vi "complementaryfilter.vi"() -> ()   [LabVIEW 2017]
uses:
  <vilib>/myRIO/Common/Instrument Driver Framework/myRIO v1.0/Encoder/typedefs/Encoder Signal Mode.ctl
  <vilib>/myRIO/Instrument Drivers/Onboard IO/Encoder/typedefs/Encoder Reference.ctl
  <vilib>/myRIO/Common/Instrument Driver Framework/Utilities/typedefs/myRIO Generic Hardware Reference.ctl
  <vilib>/myRIO/Common/Instrument Driver Framework/Utilities/typedefs/Hardware Version Enum.ctl
  <vilib>/myRIO/Common/Instrument Driver Framework/Utilities/typedefs/myRIO v1.0 Reference.ctl
  <vilib>/myRIO/Common/Instrument Driver Framework/Utilities/typedefs/Generic FPGA Reference.ctl
  <vilib>/myRIO/Common/Instrument Driver Framework/myRIO v1.0/Encoder/typedefs/Encoder Channels Enum.ctl
  <vilib>/myRIO/Common/Instrument Driver Framework/myRIO v1.0/Encoder/typedefs/Encoder Configuration v1.0.ctl
  <vilib>/userdefined/High Color/nirio_resource_hc.ctl
  <vilib>/myRIO/Common/Instrument Driver Framework/Utilities/vis/Is FPGA Ref Available.vi
  <vilib>/myRIO/Common/Instrument Driver Framework/myRIO v1.0/Encoder/vis/myRIO v1.1 Open Encoder.vi
  <vilib>/myRIO/Instrument Drivers/Onboard IO/Encoder/vis/Read.vi
  <vilib>/myRIO/Common/Instrument Driver Framework/myRIO v1.0/UART/vis/myRIO v1.0 Close UART.vi
  <vilib>/myRIO/Common/Instrument Driver Framework/Utilities/vis/Validate Channels.vi
  <vilib>/myRIO/Common/Instrument Driver Framework/myRIO v1.0/Encoder/vis/myRIO v1.0 Reserve Encoder.vi
  <vilib>/myRIO/Common/Instrument Driver Framework/myRIO v1.0/Encoder/vis/myRIO v1.0 Build MUX Configuration Encoder.vi
  <vilib>/myRIO/Common/Instrument Driver Framework/myRIO v1.0/Resource Manager/vis/myRIO v1.0 Reserve Channel List.vi
  <vilib>/myRIO/Common/Instrument Driver Framework/myRIO v1.0/Resource Manager/vis/myRIO v1.0 Create Configuration List.vi
  <vilib>/myRIO/Common/Instrument Driver Framework/myRIO v1.0/Resource Manager/vis/myRIO v1.0 Reserve Channel.vi
  <vilib>/myRIO/Common/Instrument Driver Framework/myRIO v1.0/Resource Manager/vis/myRIO v1.0 Unreserve Channel.vi
  <vilib>/myRIO/Common/Instrument Driver Framework/myRIO v1.0/Resource Manager/vis/myRIO v1.0 Build Mutex Name.vi
  <vilib>/myRIO/Common/Instrument Driver Framework/Utilities/vis/FPGA Ref Manager.vi
  <vilib>/myRIO/Common/Instrument Driver Framework/myRIO v1.0/myRIO v1.0 Reset FPGA.vi
  <vilib>/myRIO/Common/Instrument Driver Framework/myRIO v1.0/IRQ/vis/myRIO v1.0 IRQ Info FGV.vi
  <vilib>/myRIO/Common/Instrument Driver Framework/myRIO v1.0/IRQ/vis/myRIO v1.0 Timer IRQ Info FGV.vi
  <vilib>/myRIO/Common/Instrument Driver Framework/myRIO v1.0/IRQ/vis/myRIO v1.0 ISR Agent.vi
  <vilib>/Utility/VariantDataType/GetNumericInfo.vi
  <vilib>/Utility/error.llb/Error Cluster From Error Code.vi
  <vilib>/myRIO/Common/Instrument Driver Framework/myRIO v1.0/myRIO v1.1 Open.vi
  <vilib>/myRIO/Common/Instrument Driver Framework/Utilities/vis/IO Manager.vi
  <vilib>/myRIO/Common/Instrument Driver Framework/Utilities/vis/Configuration Manager.vi
  <vilib>/myRIO/Common/Instrument Driver Framework/myRIO v1.0/Resource Manager/vis/myRIO v1.0 Configure IO.vi
  <vilib>/myRIO/Common/Instrument Driver Framework/myRIO v1.0/myRIO v1.0 Close.vi
  <vilib>/myRIO/Common/Instrument Driver Framework/myRIO v1.0/Encoder/vis/myRIO v1.0 Configure Encoder.vi
  <vilib>/myRIO/Common/Instrument Driver Framework/myRIO v1.0/Encoder/vis/myRIO v1.0 Read Encoder.vi
  <vilib>/addons/control/pid/pid.llb/PID (DBL).vi
  <vilib>/myRIO/Express VI/Onboard IO/Encoder/Encoder Express VI.xnode
  <vilib>/myRIO/Instrument Drivers/Onboard IO/Encoder/vis/myRIO Encoder Open.xnode
  <vilib>/myRIO/Common/Instrument Driver Framework/myRIO v1.0/Encoder/typedefs/Encoder Count Direction Enum.ctl
  <vilib>/addons/control/pid/NI_PID_pid.lvlib
  <vilib>/myRIO/Instrument Drivers/Onboard IO/Encoder/Encoder.lvlib
  <vilib>/Analysis/NI_AALPro.lvlib
  <vilib>/robotics/Navigation/shared/WorldMap/OccupancyGridWorldMap/NI_Robotics_OccupancyGridWorldMap.lvclass
  <vilib>/myRIO/Instrument Drivers/Utilities/Utilities.lvlib
panel:
  out "x-y":dbl
  out "angle offset":dbl
  out "latest notification":dbl
  in  "stop 3":bool
  out "string":string
  out "Waveform Chart":cluster{"roll":dbl, "pitch":dbl, "yaw":dbl}(graph)
  out "yaw 2":dbl(graph)
  in  "port":refnum<visa-resource-name>="ASRL2::INSTR"
  out "XY Graph 2":cluster{dbl[], dbl[]}(graph)
  in  "stop 2":bool
  in  "Resolution":dbl=50.0
  out "Intensity Graph":dbl[][](graph)
  out "Frequency":u32=10
  in  "curPos":cluster{"x":i32, "y":i32}
  in  "endPos":cluster{"x":i32, "y":i32}={"x"=0, "y"=6}
  out "path":cluster{"X":i32, "Y":i32}[](array[cluster])
  out "Setpoint B":dbl(slide)=1.3993520911950799 scale=-10.0..10.0
  out "Setpoint A":dbl(slide)=0.6006479088049201 scale=-10.0..10.0
  out "PID B":T1(graph)={"Setpoint"=1.3993520911950799, "output"=0.10115092019020398, "dx/dt"=1.4}
  out "PID A":T1(graph)={"Setpoint"=0.6006479088049201, "output"=0.05446764760463431, "dx/dt"=0.7407999999999447}
  out "OUTPUT A":dbl(slide)=0.7407999999999447 scale=-10.0..10.0
  out "OUTPUT B":dbl(slide)=1.4 scale=-10.0..10.0
  in  "stop":bool
  in  "PID gains":T2={"proportional gain (Kc)"=0.05, "integral time (Ti, min)"=0.05, "derivative time (Td, min)"=0.0} {"derivative time (Td, min)" format="%.3f"; "integral time (Ti, min)" format="%.3f"; "proportional gain (Kc)" format="%.3f"}
  out "XY Graph":cluster{"X":dbl, "Y":dbl}[](graph)=[{"X"=3.638988671509065, "Y"=989.3451951487937}, {"X"=3.4680482195157727, "Y"=989.91873657972}]
  in  "Angle":dbl(slide) scale=-360.0..360.0
  in  "Speed":dbl(slide) scale=-10.0..10.0
  out "X, Y, BEARING 2":cluster{dbl, dbl, dbl}
  out "Final X, Y, BEARING":cluster{dbl, dbl, dbl}
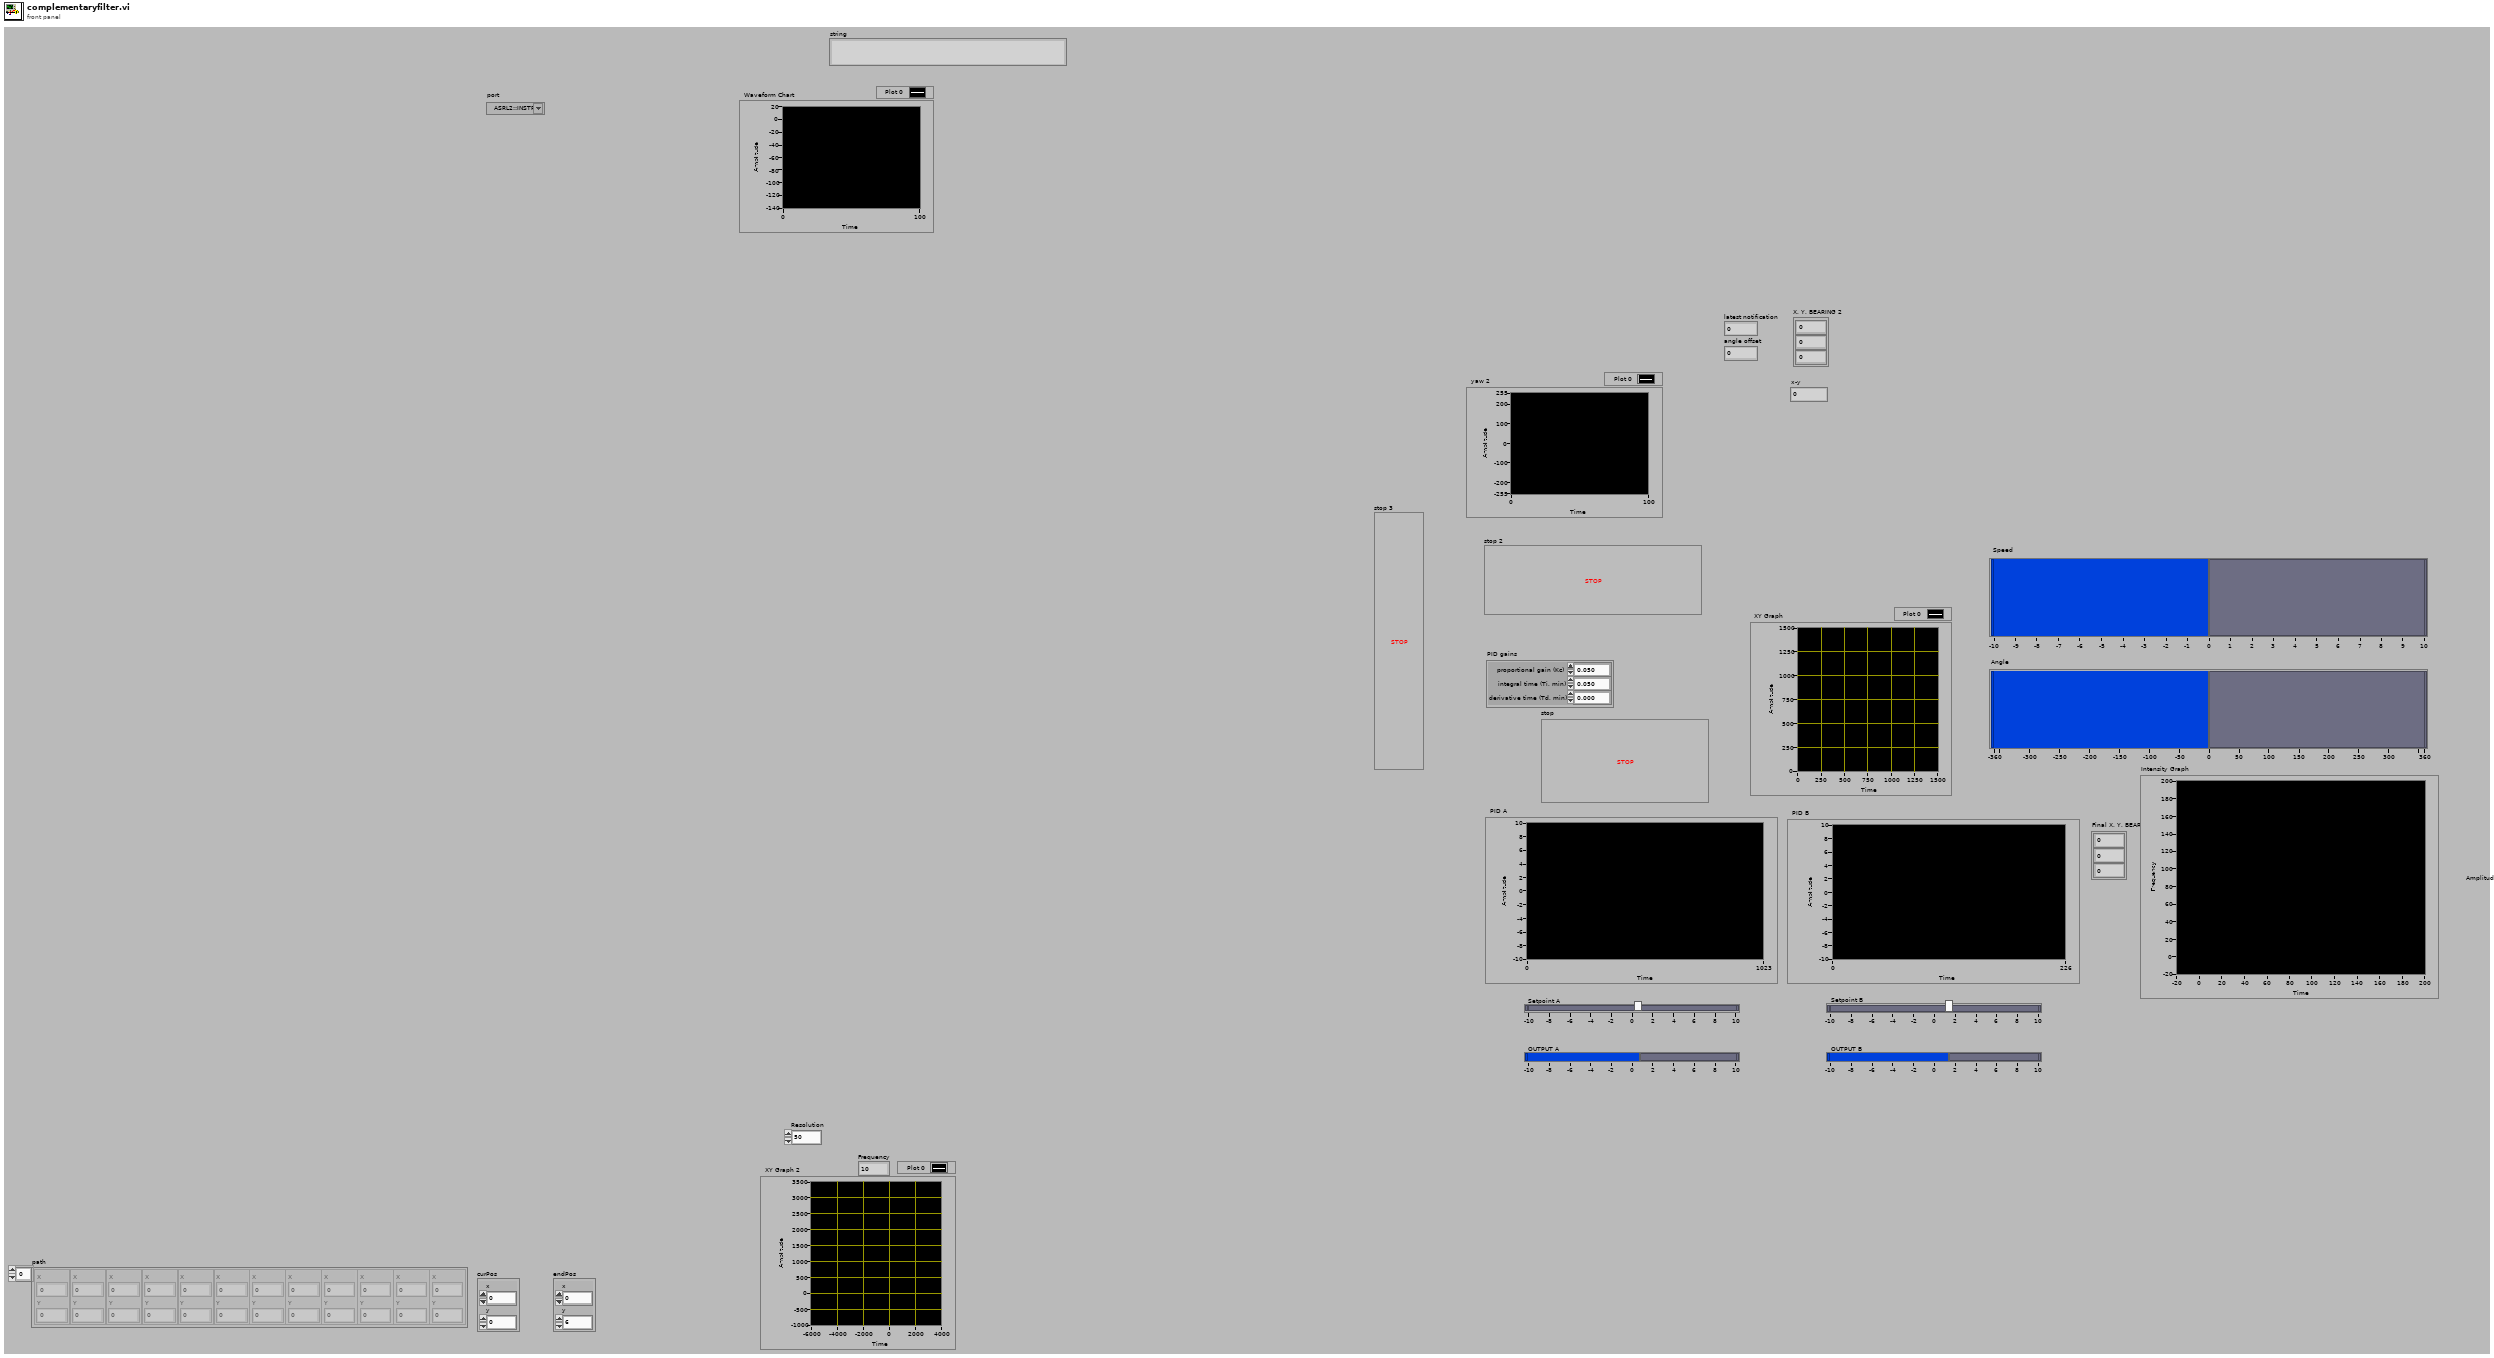
[diagram p1: front panel]
types:
  T1 = cluster{"Setpoint":dbl, "output":dbl, "dx/dt":dbl}
  T2 = cluster{"proportional gain (Kc)":dbl, "integral time (Ti, min)":dbl, "derivative time (Td, min)":dbl}
  T3 = typedef "LidarPoint.ctl" = cluster{"X":dbl, "Y":dbl}
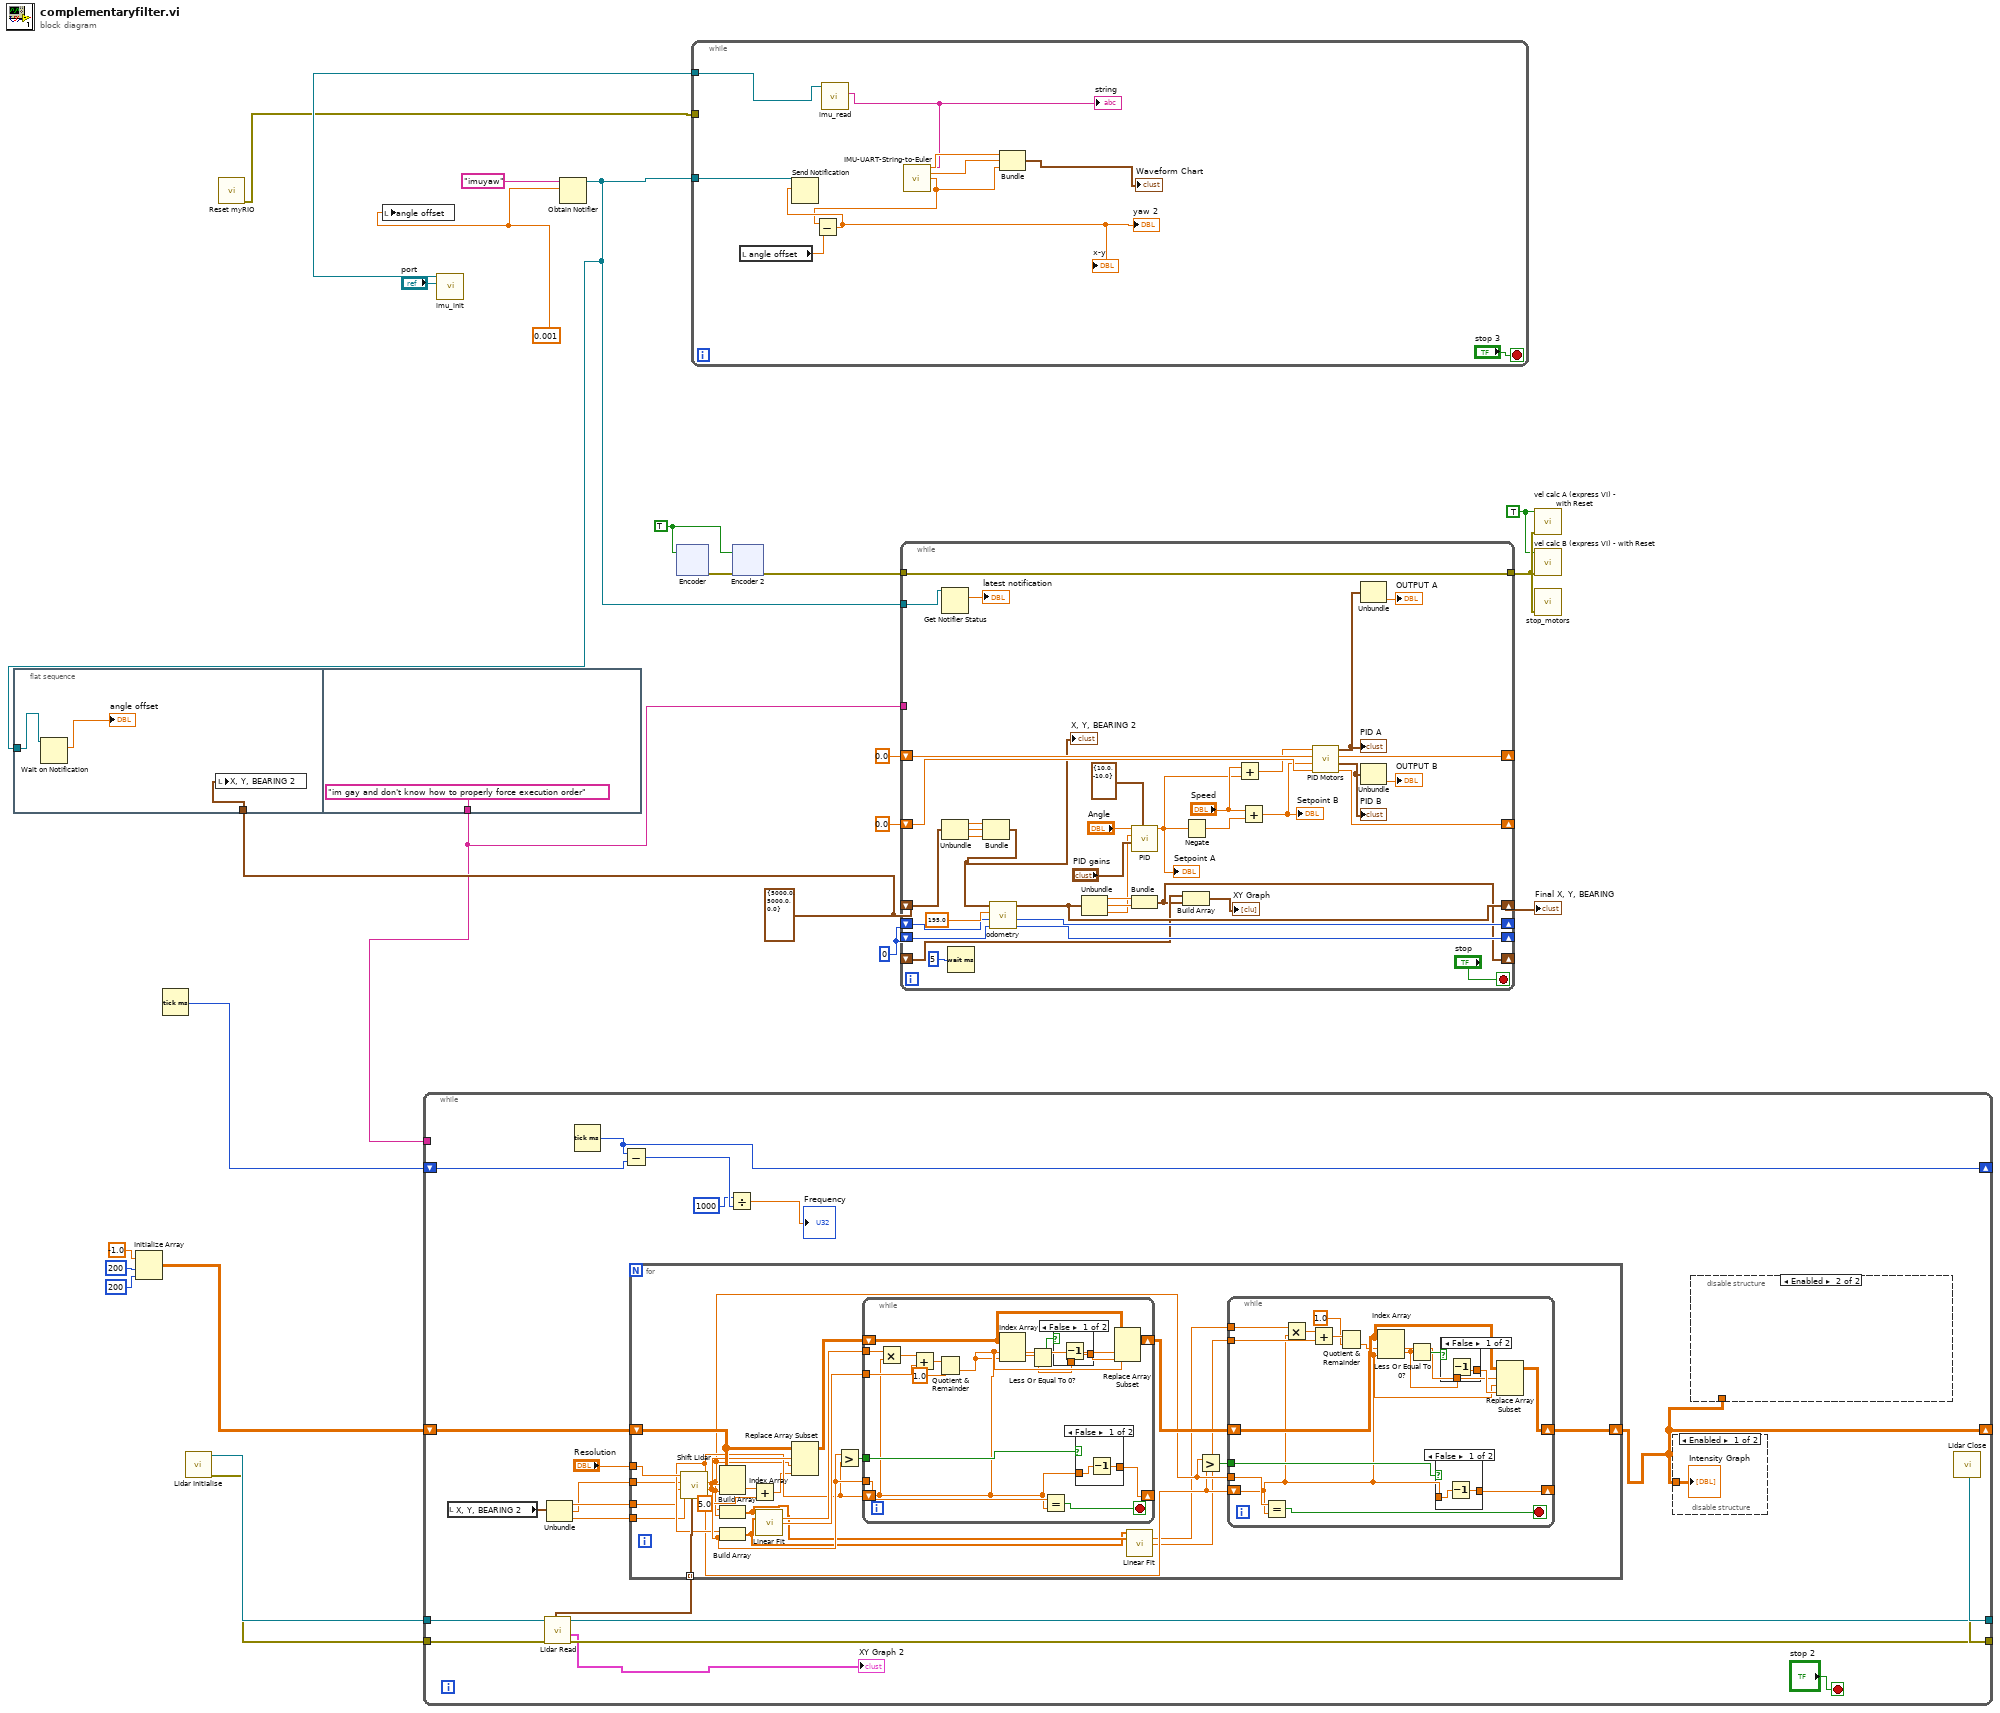
[diagram p0: block diagram]
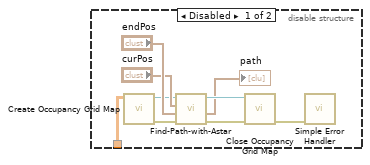
[diagram p2: hidden frame]
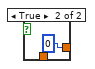
[diagram p4: hidden frame]
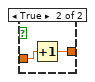
[diagram p5: hidden frame]
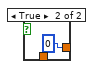
[diagram p6: hidden frame]
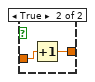
[diagram p7: hidden frame]
diagram:
  w2 = 0.001
  w8 = cluster{dbl, dbl, dbl} {5000.0, 5000.0, 0.0} ("Initial X, Y, BEARING")
  w18 = TRUE ("Reinitialise")
  w20 = TRUE
  w22 = 0 ("ENCA OUT")
  n1 = flat-sequence {
    tunnel: w8 -> [w29]
    tunnel: w3 -> [w28]
    tunnel: ["im gay and don't know how to properly force execution order"] -> w4
    frame #0 {
      n2 = Wait on Notification(notifier=w28) -> (notification=→"angle offset":dbl)  [unwired: 3 in, 3 out]
      n3 = local write "X, Y, BEARING 2"(w29) -> ()
    }
    frame #1 {
    }
  }
  n4 = Initialize Array(-1.0 ("element"), 200 ("dimension size"), 200 ("dimension size")) -> (w11:dbl[][])
  n5 = Tick Count (ms)() -> (millisecond timer value=w9:u32)
  n6 = call "Lidar Initialise.vi"() -> ("error out"=w16:errorcluster, "VISA resource name out"=w17:refnum<visa-resource-name>)  [unwired: 10 in]
  n7 = call <vilib>:"Reset myRIO.vi"() -> ("error out"=w1:errorcluster)  [unwired: 11 in]
  n8 = local write "angle offset"(w2) -> ()
  n9 = while {
    tunnel: w17 -> [w49]
    tunnel: w16 -> [w48]
    tunnel: [w47] -> w15
    tunnel: [w46] -> w14
    shift-right: [w37] -> _
    shift-left: w11 -> [w43]
    shift-right: [w40] -> _
    shift-left: w9 -> [w42]
    tunnel: w4 -> [_]
    stop <- "stop 2" stop-if-true
    n10 = local read "X, Y, BEARING 2"() -> (w34:cluster{dbl, dbl, dbl})
    n11 = call "Lidar Read.vi"("error in (no error)"=w48, "VISA resource name"=w49) -> ("error out"=w46:errorcluster, "Visual Out"=→"XY Graph 2":cluster{dbl[], dbl[]}, "VISA resource name out"=w47:refnum<visa-resource-name>, "XYflipped"=w35:T3[])  [unwired: 2 in, 3 out]
    n12 = Unbundle(w34) -> (w33:dbl, w32:dbl, w31:dbl)
    n13 = Tick Count (ms)() -> (millisecond timer value=w40:u32)
    n14 = Subtract(x=w40, y=w42) -> (x-y=w39:u32)
    n15 = for {
      tunnel: "Resolution" -> [w83]
      tunnel: w35 -> [w82] mode=indexing
      shift-right: [w70] -> w37
      shift-left: w43 -> [w81]
      tunnel: w33 -> [w62]
      tunnel: w32 -> [w61]
      tunnel: w31 -> [w60]
      n16 = call "Shift Lidar.vi"("XY"=w82, "Angle"=w60, "X position"=w62, "Y position"=w61, "Resolution"=w83) -> ("PosY"=w68:dbl, "Shifted X"=w78:dbl, "Shifted Y"=w69:dbl, "PosX"=w75:dbl)  [unwired: 3 in]
      n17 = Index Array(array=w81, index (row)=w78, index (col)=w69) -> (element=w74:dbl)
      n18 = Build Array(w68, w69) -> (w66:dbl[])
      n19 = Build Array(w75, w78) -> (w65:dbl[])
      n20 = Add(x=w74, y=5.0) -> (x+y=w73:dbl)
      n21 = call <vilib>:"Linear Fit.vi"("Y"=w66, "X"=w65) -> ("slope"=w80:dbl, "intercept"=w79:dbl)  [unwired: 9 in, 3 out]
      n22 = Replace Array Subset(array=w81, new element=w73, index (row)=w78, index (col)=w69) -> (w76:dbl[][])
      n23 = Greater?(x=w78, y=w75) -> (0:w77:bool)
      n24 = while {
        tunnel: w78 -> [w121]
        shift-right: [w119] -> _
        shift-left: w75 -> [w114]
        tunnel: w80 -> [w118]
        tunnel: w79 -> [w116]
        tunnel: w77 -> [w120]
        shift-right: [w113] -> w71
        shift-left: w76 -> [w115]
        stop <- w122 stop-if-true
        n25 = Multiply(x=w118, y=w114) -> (x*y=w117:dbl)
        n26 = Add(x=w117, y=w116) -> (x+y=w109:dbl)
        n27 = Quotient & Remainder(x=w109, y=1.0) -> (floor(x/y)=w107:dbl)  [unwired: 1 out]
        n28 = Index Array(array=w115, index (row)=w114, index (col)=w107) -> (element=w110:dbl)
        n29 = Less Or Equal To 0?(x=w110) -> (x <= 0?=w112:bool)
        n30 = Equal?(x=w121, y=w114) -> (x = y?=w122:bool)
        n31 = case shown="False" w112 {
          tunnel: [w124 0] -> w111
          tunnel: w110 -> [w123 _]
          frame False {
            n32 = Decrement(x=w123) -> (x-1=w124:dbl)
          }
          frame True {
          }
        }
        n33 = case shown="False" w120 {
          tunnel: w114 -> [w126 w129]
          tunnel: [w127 w128] -> w119
          frame False {
            n34 = Decrement(x=w126) -> (x-1=w127:dbl)
          }
          frame True {
            n35 = Increment(x=w129) -> (x+1=w128:dbl)
          }
        }
        n36 = Replace Array Subset(array=w115, new element=w111, index (row)=w114, index (col)=w107) -> (w113:dbl[][])
      }
      n37 = call <vilib>:"Linear Fit.vi"("Y"=w65, "X"=w66) -> ("slope"=w64:dbl, "intercept"=w63:dbl)  [unwired: 9 in, 3 out]
      n38 = Greater?(x=w69, y=w68) -> (0:w67:bool)
      n39 = while {
        shift-right: [w88] -> w70
        shift-left: w71 -> [w87]
        shift-right: [w96] -> _
        shift-left: w68 -> [w85]
        tunnel: w69 -> [w98]
        tunnel: w67 -> [w97]
        tunnel: w64 -> [w95]
        tunnel: w63 -> [w93]
        stop <- w99 stop-if-true
        n40 = Equal?(x=w98, y=w85) -> (x = y?=w99:bool)
        n41 = Multiply(x=w95, y=w85) -> (x*y=w94:dbl)
        n42 = Add(x=w94, y=w93) -> (x+y=w92:dbl)
        n43 = Quotient & Remainder(x=w92, y=1.0) -> (floor(x/y)=w84:dbl)  [unwired: 1 out]
        n44 = Index Array(array=w87, index (row)=w84, index (col)=w85) -> (element=w89:dbl)
        n45 = Less Or Equal To 0?(x=w89) -> (x <= 0?=w90:bool)
        n46 = case shown="False" w97 {
          tunnel: w85 -> [w103 w106]
          tunnel: [w104 w105] -> w96
          frame False {
            n47 = Decrement(x=w103) -> (x-1=w104:dbl)
          }
          frame True {
            n48 = Increment(x=w106) -> (x+1=w105:dbl)
          }
        }
        n49 = case shown="False" w90 {
          tunnel: [w101 0] -> w86
          tunnel: w89 -> [w100 _]
          frame False {
            n50 = Decrement(x=w100) -> (x-1=w101:dbl)
          }
          frame True {
          }
        }
        n51 = Replace Array Subset(array=w87, new element=w86, index (row)=w84, index (col)=w85) -> (w88:dbl[][])
      }
    }
    n52 = Divide(x=u32 1000 ("y"), y=w39) -> (x/y=→"Frequency":dbl)
    n53 = disable-structure shown="Enabled" {
      disable-tunnel: w37 -> [w59 _]
      frame Enabled {
        "Intensity Graph" <- w59
      }
      frame Disabled {
      }
    }
    n54 = disable-structure shown="Enabled" {
      disable-tunnel: w37 -> [w50 _]
      frame Disabled {
        n55 = call <vilib>:"Create Occupancy Grid Map.vi"("occupancy grid"=w50) -> ("error out"=w58:errorcluster, "map reference out"=w55:refnum<data-value>)  [unwired: 9 in]
        n56 = call "Find-Path-with-Astar.vi"("error in (no error)"=w58, "goal node"="endPos", "start node"="curPos", "map reference in"=w55) -> ("error out"=w53:errorcluster, "Array"=→"path":cluster{"X":i32, "Y":i32}[], "map reference out"=w54:refnum<data-value>)  [unwired: 5 in]
        n57 = call <vilib>:"Close Occupancy Grid Map.vi"("error in (no error)"=w53, "map reference in"=w54) -> ("error out"=w52:errorcluster)  [unwired: 9 in]
        n58 = call <vilib>:"Simple Error Handler.vi"("error in (no error)"=w52) -> ()  [unwired: 4 in, 5 out]
      }
      frame Enabled {
      }
    }
  }
  n59 = call "imu_init.vi"("port"="port") -> ("VISA resource name out"=w7:refnum<visa-resource-name>)  [unwired: 9 in, 1 out]
  n60 = Obtain Notifier(name (unnamed)="imuyaw", notification data type=w2) -> (notifier out=w3:refnum<notifier>)  [unwired: 2 in, 2 out]
  n61 = xnode "Encoder"("Reset Counter"=w20) -> ("error out"=w21:errorcluster)  [unwired: 1 in, 3 out]
  n62 = while {
    tunnel: w7 -> [w138]
    tunnel: w3 -> [w134]
    tunnel: w1 -> [_]
    stop <- "stop 3" stop-if-true
    n63 = local read "angle offset"() -> (w132:dbl)
    n64 = call "imu_read.vi"("VISA resource name"=w138) -> ("read buffer"=w133:string)  [unwired: 8 in]
    "string" <- w133
    n65 = call "IMU-UART-String-to-Euler.vi"("IMU Data"=w133) -> ("roll"=w136:dbl, "pitch"=w137:dbl, "yaw"=w130:dbl)  [unwired: 9 in, 3 out]
    n66 = Subtract(x=w130, y=w132) -> (x-y=w131:dbl)
    "yaw 2" <- w131
    "x-y" <- w131
    n67 = Send Notification(notification=w131, notifier=w134) -> ()  [unwired: 1 in, 2 out]
    n68 = Bundle("roll"=w136, "pitch"=w137, "yaw"=w130) -> (→"Waveform Chart":cluster{"roll":dbl, "pitch":dbl, "yaw":dbl})  [unwired: 1 in]
  }
  n69 = xnode "Encoder 2"("error in (no error)"=w21, "Reset Counter"=w20) -> ("error out"=w19:errorcluster)  [unwired: 3 out]
  n70 = while {
    tunnel: w19 -> [w172]
    shift-right: [w174] -> _
    shift-left: 0.0 ("output A") -> [w175]
    shift-right: [w176] -> _
    shift-left: 0.0 ("output B") -> [w151]
    tunnel: [w172] -> w25
    shift-right: [w164] -> _
    shift-left: w22 -> [w166]
    shift-right: [w163] -> _
    shift-left: w22 -> [w165]
    shift-right: [w162] -> w26
    shift-left: w8 -> [w145]
    shift-right: [w158] -> _
    shift-left: _ -> [w159]
    tunnel: w3 -> [w146]
    tunnel: w4 -> [_]
    stop <- "stop" stop-if-true
    n71 = Get Notifier Status(notifier=w146) -> (current notification=→"latest notification":dbl)  [unwired: 1 in, 4 out]
    n72 = Unbundle(w145) -> (w144:dbl, w143:dbl, w142:dbl)
    n73 = Wait (ms)(milliseconds to wait=5 ("ENCB OUT")) -> ()  [unwired: 1 out]
    n74 = Bundle(w144, w143, w142) -> (w141:cluster{dbl, dbl, dbl})  [unwired: 1 in]
    "X, Y, BEARING 2" <- w141
    n75 = call "odometry.vi"("ENCB in"=w165, "ENCA in"=w166, "wheelbase"=195.0, "Position"=w141) -> ("ENCB OUT"=w163:i32, "ENCA OUT"=w164:i32, "X, Y, BEARING"=w162:cluster{dbl, dbl, dbl})  [unwired: 4 in]
    n76 = Unbundle(w162) -> (w160:dbl, w161:dbl, w155:dbl)
    n77 = call-poly <vilib>:"PID.vi"("output range"=cluster{"output high":dbl, "output low":dbl} {"output high"=10.0, "output low"=-10.0}, "PID gains"="PID gains", "process variable"=w155, "setpoint"="Angle") -> ("output"=w148:dbl)  [unwired: 6 in, 1 out]
    "Setpoint A" <- w148
    n78 = Bundle(w160, w161) -> (w158:cluster{dbl, dbl})  [unwired: 1 in]
    n79 = Build Array(w159, w158) -> (→"XY Graph":cluster{dbl, dbl}[])
    n80 = Negate(x=w148) -> (-x=w149:dbl)
    n81 = Add(x="Speed", y=w148) -> (x+y=w147:dbl)
    n82 = Add(x="Speed", y=w149) -> (x+y=w150:dbl)
    "Setpoint B" <- w150
    n83 = call "PID Motors.vi"("input B"=w151, "Speed B"=w150, "input A"=w175, "Speed A"=w147) -> ("output B"=w176:dbl, "Speed B0"=w170:T1, "output A"=w174:dbl, "Speed A0"=w171:T1)
    "PID B" <- w170
    "PID A" <- w171
    n84 = Unbundle(w171) -> ("dx/dt"=→"OUTPUT A":dbl)  [unwired: 2 out]
    n85 = Unbundle(w170) -> ("dx/dt"=→"OUTPUT B":dbl)  [unwired: 2 out]
  }
  "Final X, Y, BEARING" <- w26
  n86 = call "vel calc A (express VI) - with Reset.vi"("error in"=w25, "Reinitialise"=w18) -> ()  [unwired: 5 in, 5 out]
  n87 = call "vel calc B (express VI) - with Reset.vi"("error in"=w25, "Reinitialise"=w18) -> ()  [unwired: 5 in, 5 out]
  n88 = call "stop_motors.vi"("error in (no error)"=w25) -> ()  [unwired: 4 in, 1 out]
  n89 = call "Lidar Close.vi"("error in (no error)"=w14, "VISA resource name"=w15) -> ()  [unwired: 9 in, 1 out]
